vi "ComplexBlob.vi"(4 "Connectivity":enum16{"4", "8"}(ring)=enum."8", 5 "Image in":T1 {"Dialogs" format="%.0b"}) -> (0 "# particles":i32, 1 "Parameters":dbl[][](array[numeric]), 2 "Image out":T1 {"Dialogs" format="%.0b"})   [LabVIEW 2024]
doc: "This VI performs a depth-first search on an image to determine the number of blobs. \n\nInput must be a binary image. \n\n<B>Connectivity</B> defines the way in which blobs are searched. 4-connectivity will yield more small blobs, since diagonals are not considered connections. 8-connectivity will yield fewer, larger blobs. \n\nOutput is an image in which each blob is identified by a number. All pixels corresponding to blob #1 are given the value 1, while all those corresponding to blob #2 are given the value 2 and so on. Also, an array of <B>blob sizes</B> indicates the number of blobs found and each of their sizes.\n\nThe Param and Position is a matrix with the first column being the parameter, the second and third columns are the X and Y locations of the centroid of the blob."
uses:
  <userlib>/ImageProcessing/QTLIB_2595_LV86/QT_Image.ctl
panel:
  # "Area"
  # "X Center   Y Center"
  # "This VI performs a depth-first search on an image to \ndetermine the number of blobs and returns a parameter\nof  the blob.\n\nInput must be a binary image.  \n\nConnectivity defines the way in which blobs are \nsearched.  4-connectivity will yield more small blobs, \nsince diagonals are not considered connections.\n8-connectivity will yield fewer, larger blobs.  \n\nOutput is an image in which each blob is identified by \na number.  All pixels corresponding to blob #1 are \ngiven the value 1, while all those corresponding to \nblob #2 are given the value 2 and so on.  Also, an array\nof blob sizes indicates the number of blobs\nfound and each of their sizes."
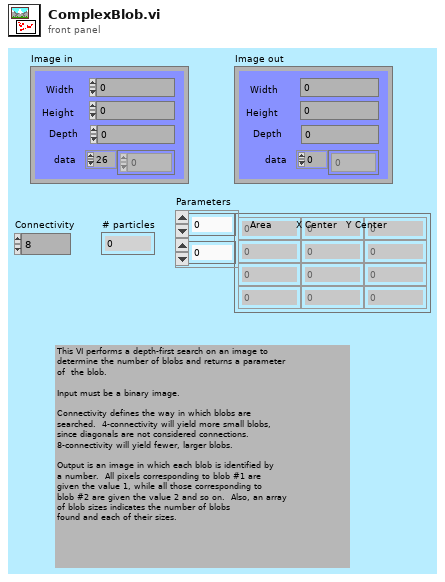
[diagram p1: front panel]
types:
  T1 = typedef "QT_Image.ctl" = cluster{"Width":i32, "Height":i32, "Depth":i32, "data":u8[], "Compressed data":u8[], "Color table":u32[], "Duration":i32, "Options":i32, "Timestamp":i32, "ID":i32, "Reserved":i32, "Dialogs":u32}
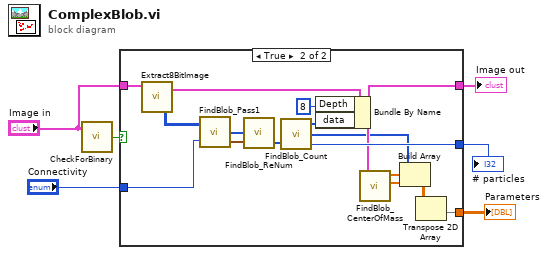
[diagram p0: block diagram]
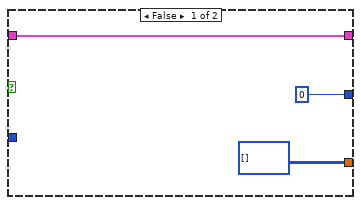
[diagram p2: hidden frame]
diagram:
  n1 = call <userlib>:"CheckForBinary.vi"("Image in"="Image in") -> ("Success?"=w6:bool)  [unwired: 2 out]
  n2 = case shown="True" w6 {
    tunnel: [w9 w17] -> w5
    tunnel: "Image in" -> [w9 w25]
    tunnel: "Connectivity" -> [_ w23]
    tunnel: [0 ("# particles") w18] -> w2
    tunnel: [i32[][] [] ("Area (pixels)") w11] -> w1
    frame False {
    }
    frame True {
      n3 = call <userlib>:"Extract8BitImage.vi"("Image in"=w25) -> ("Intensity Graph"=w24:u8[][], "Image out"=w20:T1)  [unwired: 1 in]
      n4 = call <userlib>:"FindBlob_Pass1.vi"("Image in"=w24, "Connectivity"=w23) -> ("output array"=w21:u32[], "duplicates"=w22:cluster{u8, u8, u8}[])  [unwired: 1 out]
      n5 = call <userlib>:"FindBlob_ReNum.vi"("duplicates"=w22, "Image Data in"=w21) -> ("Image Data out"=w19:u32[])
      n6 = call <userlib>:"FindBlob_Count.vi"("Image Data in"=w19) -> ("Image Data out"=w16:u32[], "Area (pixels)"=w15:i32[], "# particles"=w18:i32)  [unwired: 1 out]
      n7 = Bundle By Name(cluster=w20, "Depth"=8, "data"=w16) -> (w17:T1)
      n8 = call <userlib>:"FindBlob_CenterOfMass.vi"("Image in"=w17) -> ("center of mass Y"=w13:dbl[], "center of mass X"=w14:dbl[])  [unwired: 1 in, 3 out]
      n9 = Build Array(w15, w14, w13) -> (w12:dbl[][])
      n10 = Transpose 2D Array(2D array=w12) -> (transposed array=w11:dbl[][])
    }
  }
  "Image out" <- w5
  "Parameters" <- w1
  "# particles" <- w2
